vi "Configure Serial Bus (A429 - Autosetup).vi"(0 "VISA resource name":refnum<visa-resource-name>, 5 "Serial Bus Name (1: Serial Bus 1)":i32(ring)=1 items=["Serial Bus 1"=1, "Serial Bus 2"=2], 11 "error in (no error)":errorcluster) -> (4 "VISA resource name out":refnum<visa-resource-name>, 15 "error out":errorcluster)   [LabVIEW 2017, in "Agilent 2000 3000 X-Series.lvlib"]
doc: "Sets these options for decoding and triggering on ARINC 429 signals automatically:\nHigh Trigger Threshold: 3.0 V.\nLow Trigger Threshold: - 3.0 V.\nNoise Reject: Off.\nProbe Attenuation: 10.0.\nVertical Scale: 4 V/div.\nSerial Decode: On.\nBase: HEX.\nWord Format: LDSDi (Label/SDI/Data/SSM).\nTrigger: the specified serial bus (Serial Bus Name).\nTrigger Mode: WSTArt.\n\nNote:\nThis VI is not supported by EDUX1052A/G, DSOX1202A/G, DSOX1204A/G models"
uses:
  Agilent 2000 3000 X-Series.lvlib
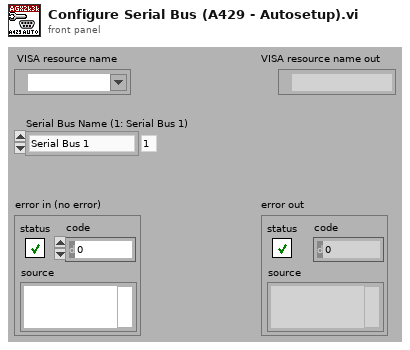
[diagram p1: front panel]
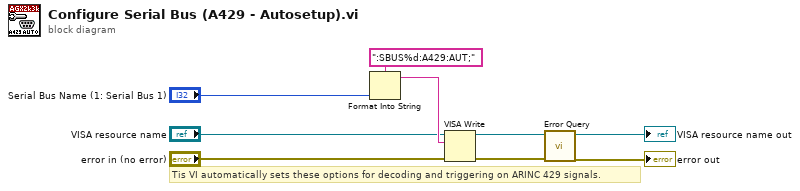
[diagram p0: block diagram]
diagram:
  # "Tis VI automatically sets these options for decoding and triggering on ARINC 429 signals."
  n1 = Format Into String(format string=":SBUS%d:A429:AUT;", "Serial Bus Name (1: Serial Bus 1)") -> (resulting string=w7:string)  [unwired: 2 in, 1 out]
  n2 = VISA Write(VISA resource name="VISA resource name", write buffer=w7, error in (no error)="error in (no error)") -> (VISA resource name out=w4:refnum<visa-resource-name>, error out=w3:errorcluster)  [unwired: 1 out]
  n3 = call "Error Query.vi"("error in (no error)"=w3, "VISA resource name"=w4) -> ("error out"=→"error out":errorcluster, "VISA resource name out"=→"VISA resource name out":refnum<visa-resource-name>)  [unwired: 8 out]
